vi "Reconstitution face (SubVI).vi"(0 "Couleur carrée  2":string[](array[string]), 1 "Couleur carrée  1":string[](array[string]), 2 "Couleur carrée 0":string[](array[string]), 5 "Couleur carrée  3":string[](array[string]), 7 "Couleur carrée  5":string[](array[string]), 9 "Couleur carrée  6":string[](array[string]), 11 "Couleur carrée  7":string[](array[string]), 12 "Couleur carrée  8":string[](array[string])) -> (3 "Couleur 0":string, 4 "Couleur 1":string, 6 "Couleur  2":string, 8 "Couleur 3":string, 10 "Couleur 5":string, 13 "Couleur 8":string, 14 "Couleur 7":string, 15 "Couleur 6":string)   [LabVIEW 2019]
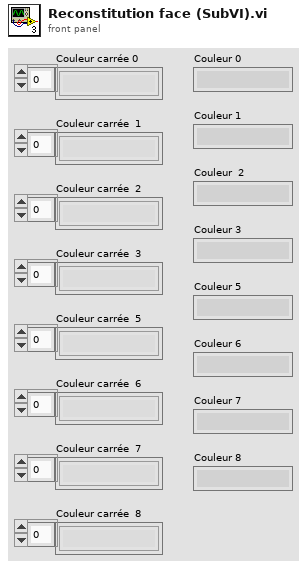
[diagram p1: front panel]
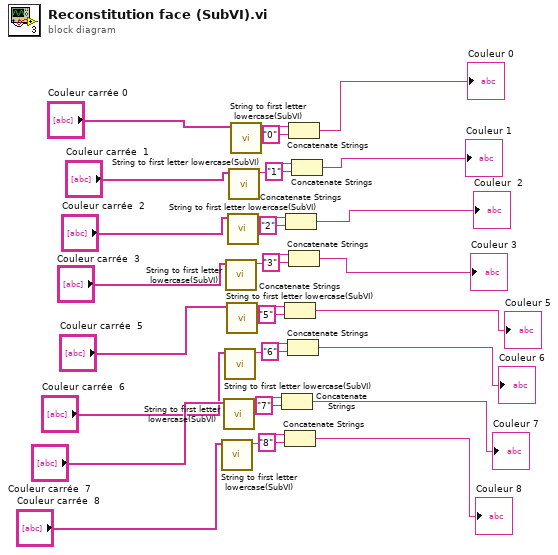
[diagram p0: block diagram]
diagram:
  n1 = call "String to first letter lowercase(SubVI).vi"("Couleur carré"="Couleur carrée  8") -> ("String"=w12:string)  [unwired: 10 in]
  n2 = call "String to first letter lowercase(SubVI).vi"("Couleur carré"="Couleur carrée  7") -> ("String"=w9:string)  [unwired: 10 in]
  n3 = call "String to first letter lowercase(SubVI).vi"("Couleur carré"="Couleur carrée  6") -> ("String"=w13:string)  [unwired: 10 in]
  n4 = call "String to first letter lowercase(SubVI).vi"("Couleur carré"="Couleur carrée  3") -> ("String"=w5:string)  [unwired: 10 in]
  n5 = call "String to first letter lowercase(SubVI).vi"("Couleur carré"="Couleur carrée  5") -> ("String"=w16:string)  [unwired: 10 in]
  n6 = call "String to first letter lowercase(SubVI).vi"("Couleur carré"="Couleur carrée  2") -> ("String"=w8:string)  [unwired: 10 in]
  n7 = call "String to first letter lowercase(SubVI).vi"("Couleur carré"="Couleur carrée  1") -> ("String"=w4:string)  [unwired: 10 in]
  n8 = call "String to first letter lowercase(SubVI).vi"("Couleur carré"="Couleur carrée 0") -> ("String"=w1:string)  [unwired: 10 in]
  n9 = Concatenate Strings(w9, "7" ("string")) -> (→"Couleur 7":string)
  n10 = Concatenate Strings(w16, "5" ("string")) -> (→"Couleur 5":string)
  n11 = Concatenate Strings(w12, "8" ("string")) -> (→"Couleur 8":string)
  n12 = Concatenate Strings(w8, "2" ("string")) -> (→"Couleur  2":string)
  n13 = Concatenate Strings(w13, "6" ("string")) -> (→"Couleur 6":string)
  n14 = Concatenate Strings(w1, "0" ("string")) -> (→"Couleur 0":string)
  n15 = Concatenate Strings(w5, "3" ("string")) -> (→"Couleur 3":string)
  n16 = Concatenate Strings(w4, "1" ("string")) -> (→"Couleur 1":string)
